vi "剖面启动选择.vi"() -> (3 "check？":bool)   [LabVIEW 2016, in "main.lvlib"]
uses:
  main.lvlib
panel:
  in  "取消":bool
  in  "确定":bool
  in  "测试表层":bool
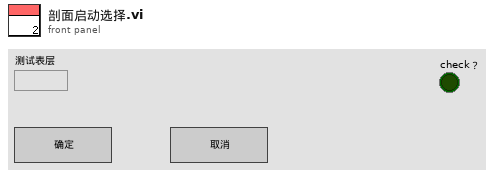
[diagram p1: front panel]
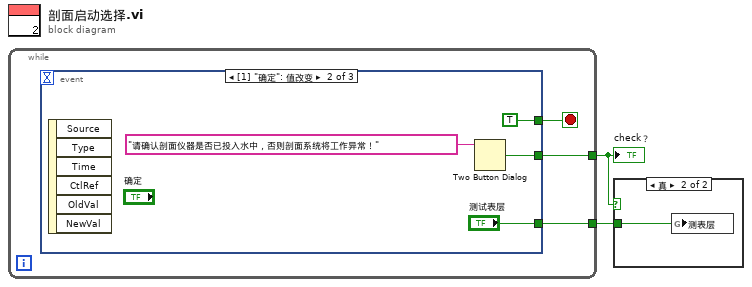
[diagram p0: block diagram]
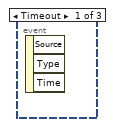
[diagram p3: hidden frame]
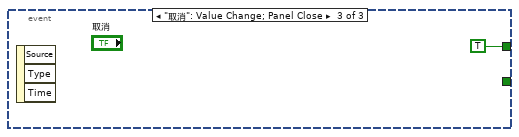
[diagram p4: hidden frame]
diagram:
  n1 = while {
    tunnel: [w4] -> w2
    tunnel: [w3] -> w1
    stop <- w5 stop-if-true
    n2 = event shown="[1] \"确定\": 值改变" {
      selector: _ -> [_ _ _]
      dyn-events: _ -> [_ _ _]
      timeout: _ -> [_ _ _]
      tunnel: [_ TRUE TRUE] -> w5
      tunnel: [_ w7 _] -> w4
      tunnel: [_ "测试表层" _] -> w3
      event Timeout {
        n3 = event-data() -> ()  [unwired: 1 in, 3 out]
      }
      event "确定": Value Change {
        n4 = event-data() -> ()  [unwired: 1 in, 6 out]
        n5 = Two Button Dialog(message="请确认剖面仪器是否已投入水中，否则剖面系统将工作异常！" ("消息")) -> (T button?=w7:bool)  [unwired: 2 in]
      }
      event "取消": Value Change; Panel Close {
        n6 = event-data() -> ()  [unwired: 1 in, 3 out]
      }
    }
  }
  "check？" <- w2
  n7 = case shown="真" w2 {
    tunnel: w1 -> [_ w11]
    frame False {
    }
    frame True {
      n8 = global write "全局非断电保持变量.vi" "测表层"(w11) -> ()
    }
  }
